vi "OFDM_FrequencyOffsetEstimation(CP).vi"(10 "sampling period":dbl format="%#_13g", 11 "input OFDM symbol":cdb[](array[numeric])) -> (3 "output OFDM symbol":cdb[](array[numeric]))   [LabVIEW 2018]
uses:
  <vilib>/Analysis/baseanly.llb/Mean (DBL).vi
  <vilib>/Analysis/NI_AALBase.lvlib
panel:
  out "Waveform Graph":dbl[](graph)
  out "frequency offset(CP)":dbl
  out "Waveform Graph 2":dbl[](graph)
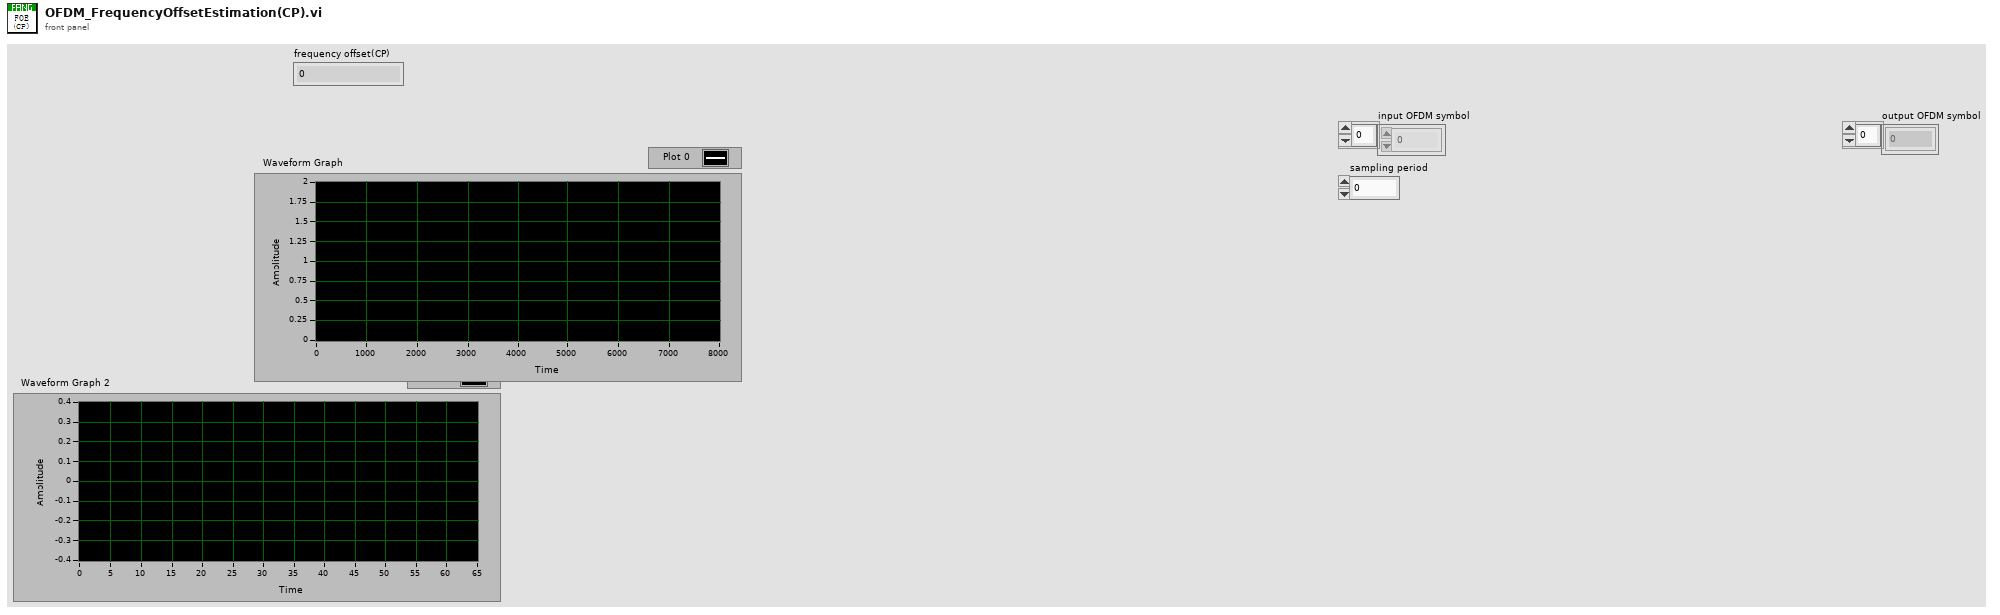
[diagram p1: front panel]
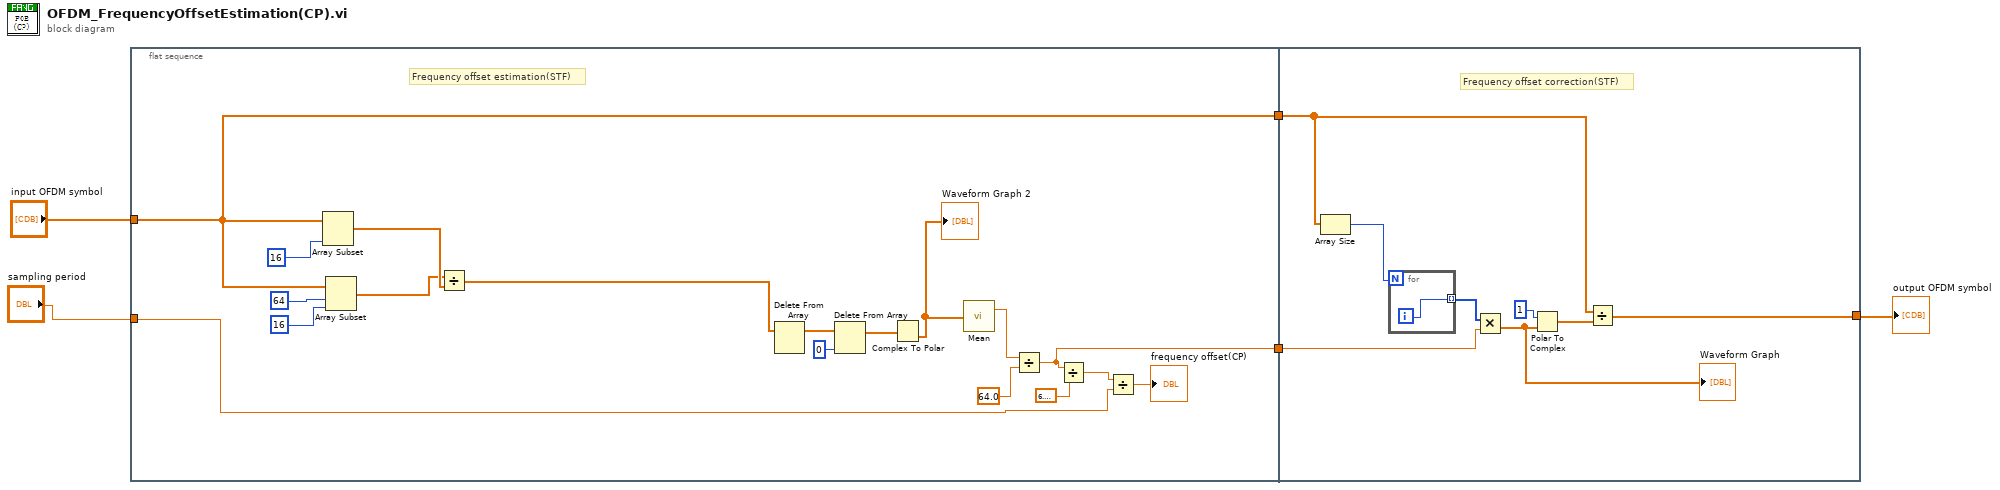
[diagram p0: block diagram]
diagram:
  n1 = flat-sequence {
    tunnel: [w7] -> w5
    tunnel: [w18] -> w4
    tunnel: "input OFDM symbol" -> [w7]
    tunnel: "sampling period" -> [w6]
    tunnel: w5 -> [w26]
    tunnel: w4 -> [w25]
    tunnel: [w24] -> w1
    frame #0 {
      # "Frequency offset estimation(STF)"
      n2 = Array Subset(array=w7, length=16) -> (w11:cdb[])  [unwired: 1 in]
      n3 = Array Subset(array=w7, index=64, length=16) -> (w10:cdb[])
      n4 = Divide(x=w10, y=w11) -> (x/y=w12:cdb[])
      n5 = Delete From Array(array=w12) -> (array with subset deleted=w13:cdb[])  [unwired: 2 in, 1 out]
      n6 = Delete From Array(array=w13, index=0) -> (array with subset deleted=w9:cdb[])  [unwired: 1 in, 1 out]
      n7 = Complex To Polar(r * e^(i*theta)=w9) -> (theta=w8:dbl[])  [unwired: 1 out]
      "Waveform Graph 2" <- w8
      n8 = call-poly <vilib>:"Mean.vi"("X"=w8) -> ("mean"=w19:dbl)  [unwired: 1 out]
      n9 = Divide(x=w19, y=64.0) -> (x/y=w18:dbl)
      n10 = Divide(x=w18, y=6.283185307179586) -> (x/y=w21:dbl)
      n11 = Divide(x=w21, y=w6) -> (x/y=→"frequency offset(CP)":dbl)
    }
    frame #1 {
      # "Frequency offset correction(STF)"
      n12 = Array Size(array=w26) -> (size(s)=w28:i32)
      n13 = for {
        N: w28 -> [_]
        tunnel: [w32] -> w27 mode=indexing
        i -> [w32]
      }
      n14 = Multiply(x=w27, y=w25) -> (x*y=w31:dbl[])
      "Waveform Graph" <- w31
      n15 = Polar To Complex(1:w31, 2:1) -> (0:w30:cdb[])
      n16 = Divide(x=w26, y=w30) -> (x/y=w24:cdb[])
    }
  }
  "output OFDM symbol" <- w1
